vi "autonTurn.vi"(8 "safety switch":bool, 9 "setpoint":dbl format="%.2f", 10 "navX Device":T1={"Interface"={"Protocol"=enum."SERIAL", "Update Rate (4Hz-60Hz)"=4, "navX Open TypeDef"=variant}, "Notify Packet"=refnum, "Loop VI Refnum"=refnum, "Ready to Close Occurrence Refnum"=refnum} {"Interface"."Update Rate (4Hz-60Hz)" min=4 max=60 step=1}, 11 "RobotDriveDevRef 2":T3={"DevStatus"={"status"=FALSE, "code"=0, "source"=""}, "Motors[]"=[], "Square Inputs"=FALSE, "Max Output"=1.0}) -> (1 "end":bool, 2 "navX Device 2":T1={"Interface"={"Protocol"=enum."SERIAL", "Update Rate (4Hz-60Hz)"=4, "navX Open TypeDef"=variant}, "Notify Packet"=refnum, "Loop VI Refnum"=refnum, "Ready to Close Occurrence Refnum"=refnum} {"Interface"."Update Rate (4Hz-60Hz)" min=4 max=60 step=1}, 3 "RobotDriveDevRef":T3={"DevStatus"={"status"=FALSE, "code"=0, "source"=""}, "Motors[]"=[], "Square Inputs"=FALSE, "Max Output"=1.0})   [LabVIEW 2015]
uses:
  <vilib>/Rock Robotics/WPI/RobotDrive/WPI_RobotDriveDevRef.ctl
  <vilib>/Rock Robotics/WPI/MotorControl/WPI_MotorControlDeviceRef.ctl
  <vilib>/Rock Robotics/WPI/MotorControl/WPI_MotorControlType.ctl
  <vilib>/Rock Robotics/SystemInterfaces/DIO/FPGA_DIOPWMChannel.ctl
  <vilib>/Rock Robotics/WPI/PWM/WPI_PWMDeadband.ctl
  <vilib>/Rock Robotics/WPI/CAN/Jaguar/SubVIs/WPI_CANJaguar_ControlMode.ctl
  <vilib>/Rock Robotics/WPI/CAN/TalonSRX/WPI_CANTalonSRX_APIControlMode.ctl
  navX-MXP-LabVIEW/navX Library v2/TypeDefs/Z900_navX_DeviceTypeDef.ctl
  navX-MXP-LabVIEW/navX Library v2/TypeDefs/Z900_navX_ProtocolTypeDef.ctl
  navX-MXP-LabVIEW/navX Library v2/TypeDefs/Z900_navX_NotifyPacketTypeDef.ctl
  navX-MXP-LabVIEW/navX Library v2/TypeDefs/Z900_navX_ActionTypeDef.ctl
  <vilib>/addons/control/pid/pid.llb/PID (DBL).vi
  <vilib>/addons/control/pid/NI_PID_pid.lvlib
  navX-MXP-LabVIEW/navX Library v2/navX Library v2.lvlib
  <vilib>/Rock Robotics/WPI/RobotDrive/WPI_RobotDriveArcadeDrive_Standard(NoSaturation).vi
panel:
  out "Yaw":dbl(graph)
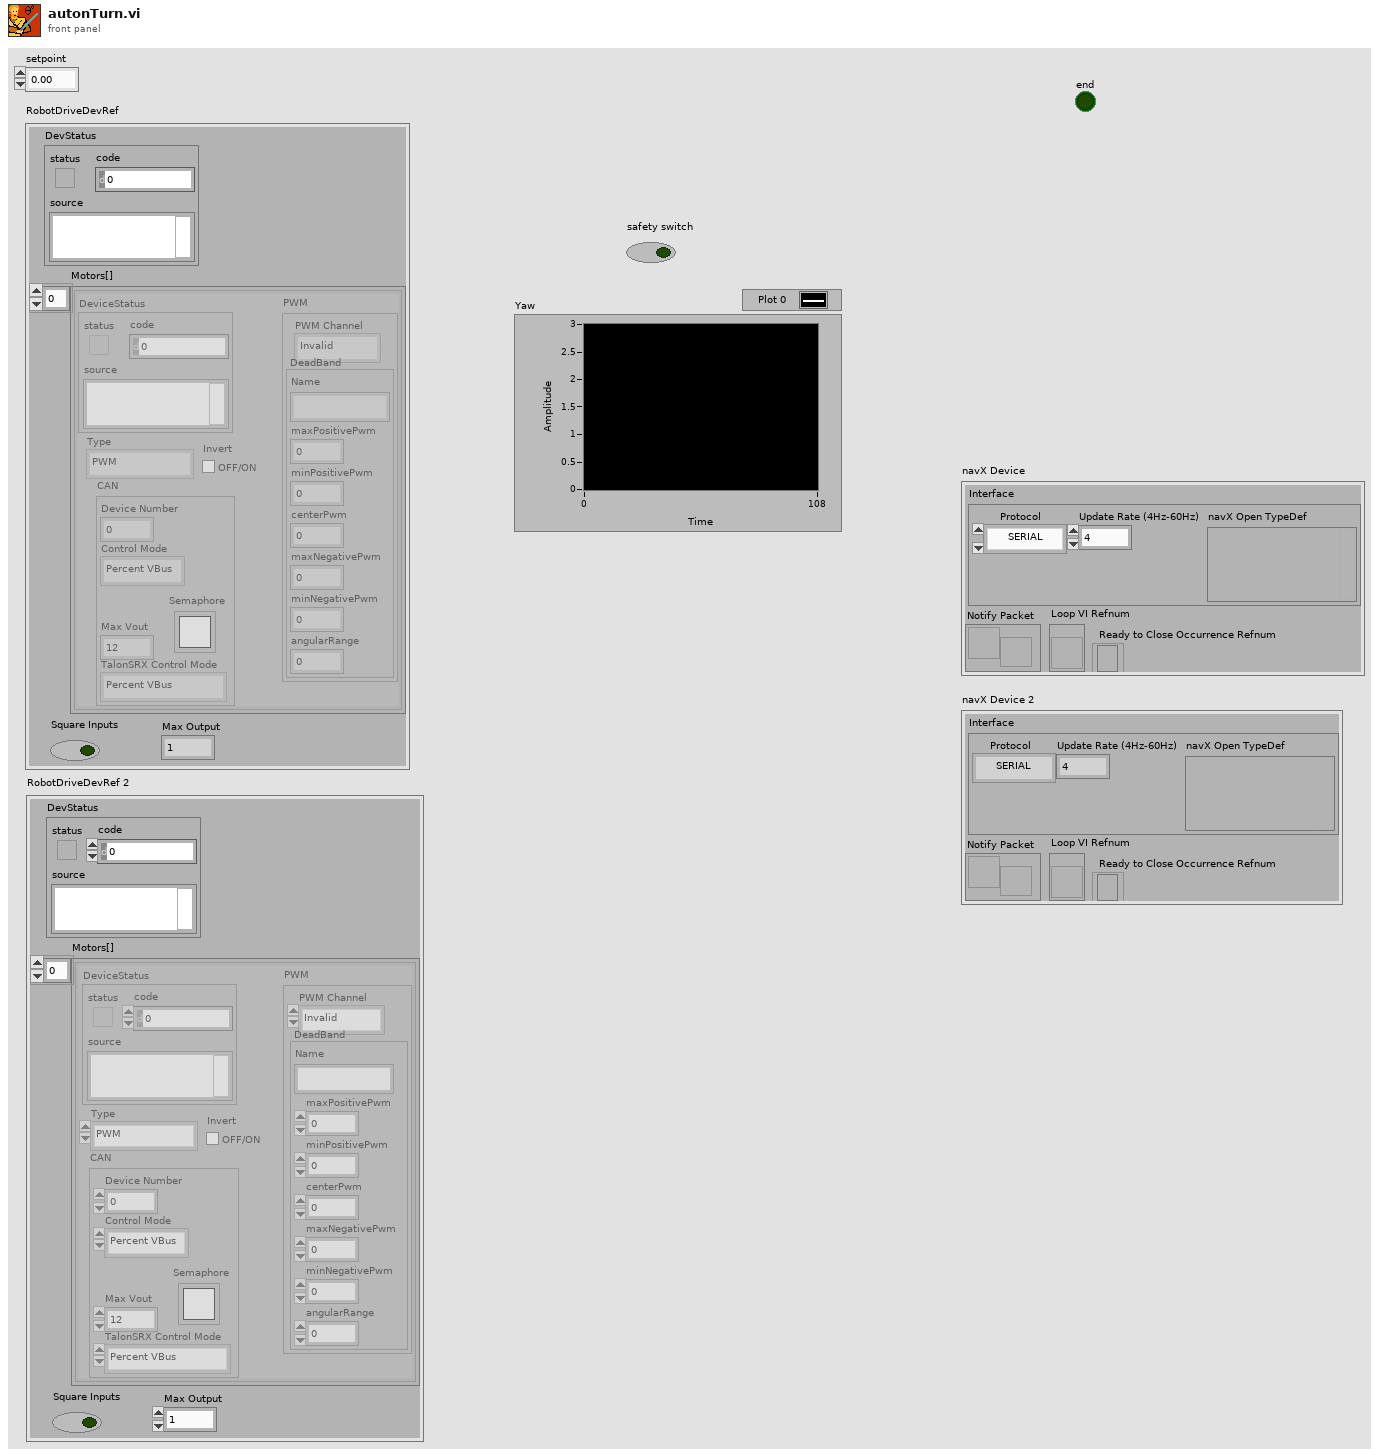
[diagram p1: front panel]
types:
  T1 = typedef "navX Library v2.lvlib/Z900_navX_DeviceTypeDef.ctl" = cluster{"Interface":cluster{"Protocol":T2, "Update Rate (4Hz-60Hz)":u8, "navX Open TypeDef":variant}, "Notify Packet":refnum<notifier>, "Loop VI Refnum":refnum<vi>, "Ready to Close Occurrence Refnum":refnum<k4>}
  T2 = typedef "navX Library v2.lvlib/Z900_navX_ProtocolTypeDef.ctl" = enum16{"SERIAL", "I2C", "SPI"}
  T3 = typedef "WPI_RobotDriveDevRef.ctl" = cluster{"DevStatus":errorcluster, "Motors[]":T4[], "Square Inputs":bool, "Max Output":dbl}
  T4 = typedef "WPI_MotorControlDeviceRef.ctl" = cluster{"DeviceStatus":errorcluster, "Type":T5, "PWM":cluster{"PWM Channel":T6, "DeadBand":T7}, "CAN":cluster{"Device Number":u8, "Control Mode":T8, "Semaphore":T9, "Max Vout":dbl, "TalonSRX Control Mode":T10}, "Invert":bool}
  T5 = typedef "WPI_MotorControlType.ctl" = enum16{"PWM", "CAN", "CANTalonSRX"}
  T6 = typedef "FPGA_DIOPWMChannel.ctl" = enum8{"PWM 0", "PWM 1", "PWM 2", "PWM 3", "PWM 4", "PWM 5", "PWM 6", "PWM 7", "PWM 8", "PWM 9", "PWM MXP 0", "PWM MXP 1", "PWM MXP 2", "PWM MXP 3", "PWM MXP 4", "PWM MXP 5", "PWM MXP 6", "PWM MXP 7", "PWM MXP 8", "PWM MXP 9", "Invalid"}
  T7 = typedef "WPI_PWMDeadband.ctl" = cluster{"Name":string, "maxPositivePwm":i32, "minPositivePwm":i32, "centerPwm":i32, "maxNegativePwm":i32, "minNegativePwm":i32, "angularRange":u16}
  T8 = typedef "WPI_CANJaguar_ControlMode.ctl" = enum8{"Percent VBus", "Current", "Speed", "Position", "Voltage"}
  T9 = typedef "Semaphore RefNum" = refnum<k1>
  T10 = typedef "WPI_CANTalonSRX_APIControlMode.ctl" = enum8{"Percent VBus", "Speed", "Position", "Slave", "Unchanged / Invalid", "Voltage Compensation", "Current", "Motion Profile"}
  T11 = cluster{"proportional gain (Kc)":dbl, "integral time (Ti, min)":dbl, "derivative time (Td, min)":dbl}
  T12 = cluster{"Yaw":dbl, "Roll":dbl, "Pitch":dbl, "Heading":dbl, "Fused Heading":dbl}
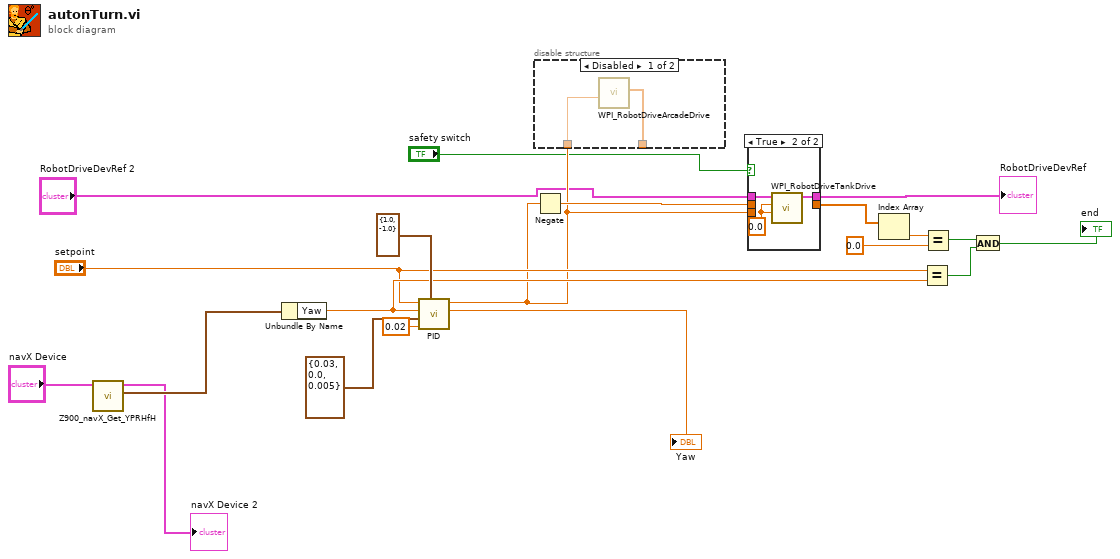
[diagram p0: block diagram]
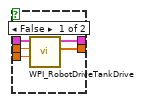
[diagram p2: hidden frame]
diagram:
  n1 = call "Z900_navX_Get_YPRHfH.vi"("navX Device"="navX Device") -> ("YRPHfH"=w10:T12, "navX Device"=→"navX Device 2":T1)  [unwired: 7 in, 2 out]
  n2 = Unbundle By Name(w10) -> ("Yaw"=w17:dbl)
  "Yaw" <- w17
  n3 = call-poly <vilib>:"PID.vi"("output range"=cluster{"output high":dbl, "output low":dbl} {"output high"=1.0, "output low"=-1.0}, "dt (s)"=0.02, "PID gains"=T11 {"proportional gain (Kc)"=0.03, "integral time (Ti, min)"=0.0, "derivative time (Td, min)"=0.005}, "process variable"=w17, "setpoint"="setpoint") -> ("output"=w6:dbl)  [unwired: 5 in, 1 out]
  n4 = disable-structure shown="Disabled" {
    disable-tunnel: w6 -> [w21 _]
    disable-tunnel: [w20 _] -> _
    frame Disabled {
      n5 = call-poly <vilib>:"WPI_RobotDriveArcadeDrive.vi"("Y axis value"=w21) -> ("Motor Values"=w20:dbl[])  [unwired: 8 in, 2 out]
    }
    frame Enabled {
    }
  }
  n6 = Negate(x=w6) -> (-x=w7:dbl)
  n7 = case shown="True" "safety switch" {
    tunnel: w7 -> [w26 _]
    tunnel: w6 -> [w25 _]
    tunnel: "RobotDriveDevRef 2" -> [w24 w29]
    tunnel: [w23 w28] -> w4
    tunnel: [w22 _] -> w3
    frame False {
      n8 = call <vilib>:"WPI_RobotDriveTankDrive.vi"("Right axis value"=w25, "Left axis value"=w26, "RobotDriveDevRef"=w24) -> ("Motor Values"=w22:dbl[], "RobotDriveDevRef"=w23:T3)  [unwired: 6 in, 1 out]
    }
    frame True {
      w27 = 0.0 ("Right axis value")
      n9 = call <vilib>:"WPI_RobotDriveTankDrive.vi"("Right axis value"=w27, "Left axis value"=w27, "RobotDriveDevRef"=w29) -> ("RobotDriveDevRef"=w28:T3)  [unwired: 6 in, 2 out]
    }
  }
  "RobotDriveDevRef" <- w4
  n10 = Index Array(array=w3) -> (element=w15:dbl)  [unwired: 1 in]
  n11 = Equal?(x="setpoint", y=w17) -> (x = y?=w12:bool)
  n12 = Equal?(x=w15, y=0.0) -> (x = y?=w13:bool)
  n13 = And(x=w13, y=w12) -> (x .and. y?=→"end":bool)
